vi "SQL_Table_Unit_Test_insert.vi"(9 "数据数值":dbl, 10 "数据名称":string, 11 "时间标识":timestamp) -> (3 "error out":errorcluster)   [LabVIEW 2014]
uses:
  Terminal_Global_TestID.vi
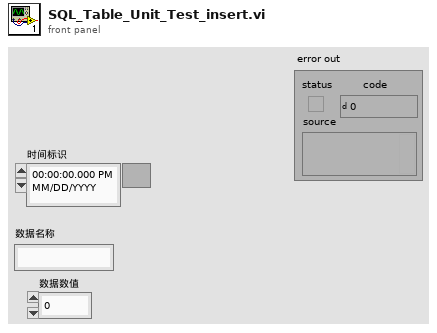
[diagram p1: front panel]
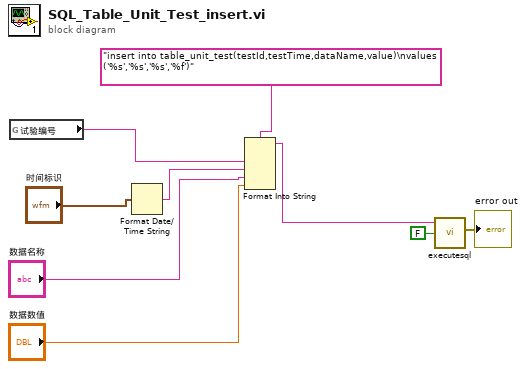
[diagram p0: block diagram]
diagram:
  n1 = global read "Terminal_Global_TestID.vi" "试验编号"() -> (w1:string)
  n2 = Format Date/Time String(seconds (now)="时间标识") -> (date/time string=w7:string)  [unwired: 2 in]
  n3 = Format Into String(format string="insert into table_unit_test(testId,testTime,dataName,value)\nvalues ('%s','%s','%s','%f')", w1, w7, "数据名称", "数据数值") -> (resulting string=w4:string)  [unwired: 2 in, 1 out]
  n4 = call "executesql.vi"("Return Data (T)"=FALSE, "Command Text"=w4) -> ("error out"=→"error out":errorcluster)  [unwired: 5 in, 1 out]
